vi "BuildingSingleImageGreyLevelDataBase.vi"(6 "Running Index":i32, 8 "error in (no error)":errorcluster, 9 "ConfDB":T1={"NumberOfImages"=0, "NoImages2SaveAroundFreeze"=0, "Path"=path "", "NameOfPartialFile"="", "StartIndex"=0, "NumberOfStdTol"=0, "Detla t (sec)"=0, "Number of images for baseline"=10, "Temperature File Name"="", "Score"=15.0, "Index number of Files"=[], "End Index"=2187}, 10 "Droplet Bounding Box":cluster{"x":sgl, "y":sgl}[][](array[cluster]), 11 "Image Ref In":T2) -> (0 "error out":errorcluster, 1 "Difference in Grey Level":dbl[](array[numeric]), 2 "GreyLevelArray":dbl[](array[numeric]))   [LabVIEW 2013]
doc: "Go over all images and retrieve Grey level of each drop and the difference between the i+1 and i image"
uses:
  <vilib>/vision/Image Controls.llb/IMAQ Image.ctl
  DB/ConfDB.ctl
  DB/DbEnum.ctl
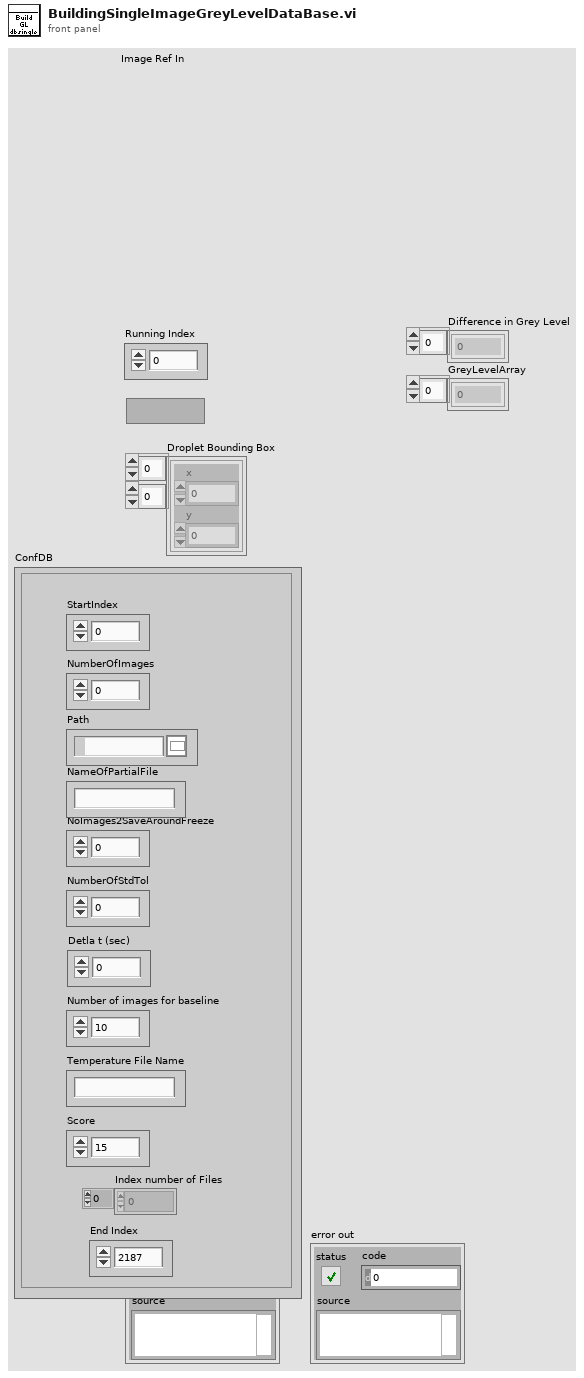
[diagram p1: front panel]
types:
  T1 = typedef "ConfDB.ctl" = cluster{"NumberOfImages":i32, "NoImages2SaveAroundFreeze":i32, "Path":path, "NameOfPartialFile":string, "StartIndex":i32, "NumberOfStdTol":i32, "Detla t (sec)":i32, "Number of images for baseline":i32, "Temperature File Name":string, "Score":dbl, "Index number of Files":i32[], "End Index":i32}
  T2 = typedef "IMAQ Image.ctl" = refnum<image>
  T3 = typedef "DbEnum.ctl" = enum16{"Write DropletDB", "Init", "Insert Detection Result Data", "Insert Grey Level Result", "Insert Baseline Results", "AddFreezeImagesAtCertainDroplet", "UpdateIncludeDroplet", "Insert Freeze Analysis Results", "GetDropDB", "GetNoFreezedDroplets", "GetGreyLevelAndDiff", "GetGreyLevelatIndexTime", "GetDropletsBoundingBox"}
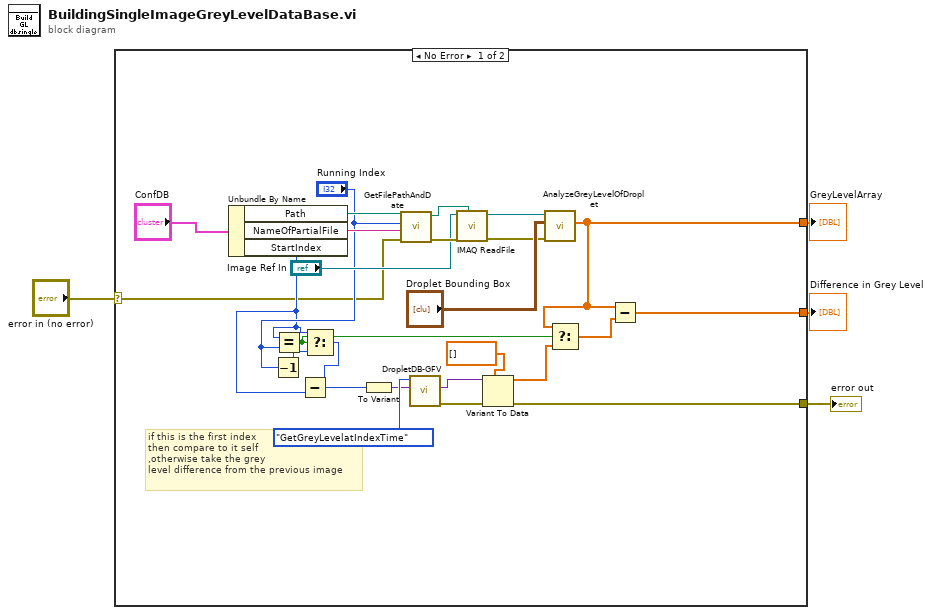
[diagram p0: block diagram]
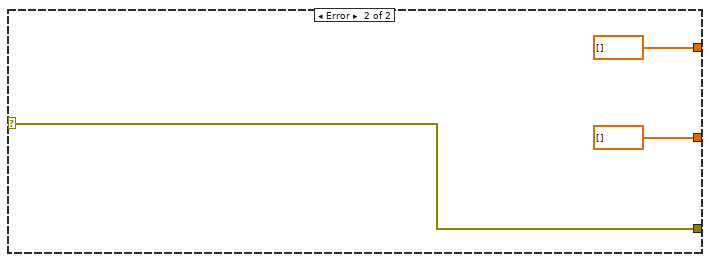
[diagram p2: hidden frame]
diagram:
  n1 = case shown="No Error" "error in (no error)" {
    selector: "error in (no error)" -> [w7 w33]
    tunnel: [w5 w33] -> w3
    tunnel: [w22 dbl[] []] -> w2
    tunnel: [w11 dbl[] [] ("GreyLevelArray")] -> w1
    frame No Error {
      # "if this is the first index\nthen compare to it self\n,otherwise take the grey\nlevel difference from the previous image"
      n2 = Unbundle By Name("ConfDB") -> ("Path"=w25:path, "NameOfPartialFile"=w26:string, "StartIndex"=w14:i32)
      n3 = Decrement(x="Running Index") -> (x-1=w23:i32)
      n4 = Equal?(x=w14, y="Running Index") -> (x = y?=w12:bool)
      n5 = Select(t=w14, s=w12, f=w23) -> (s? t:f=w17:i32)
      n6 = Subtract(x=w17, y=w14) -> (x-y=w13:i32)
      n7 = To Variant(anything=w13) -> (Variant=w18:variant)
      n8 = call "GetFilePathAndDate.vi"("error in (no error)"=w7, "String"=w26, "Index"="Running Index", "Path"=w25) -> ("error out"=w30:errorcluster, "file out"=w8:path)  [unwired: 5 in, 1 out]
      n9 = call "DropletDB-GFV.vi"("Data in"=w18, "Command In"=DbEnum."GetGreyLevelatIndexTime") -> ("error out"=w20:errorcluster, "Data out"=w19:variant)  [unwired: 8 in]
      n10 = call "IMAQ ReadFile"("File Path"=w8, "error in (no error)"=w30, "Image"="Image Ref In") -> ("error out"=w6:errorcluster, "Image Out"=w27:T2)  [unwired: 2 in, 5 out]
      n11 = Variant To Data(error in=w20, type=dbl[] [] ("GreyLevelArray"), Variant=w19) -> (data=w10:dbl[], error out=w5:errorcluster)
      n12 = call "AnalyzeGreyLevelOfDroplet.vi"("error in (no error)"=w6, "Bounding Box"="Droplet Bounding Box", "Image In"=w27) -> ("GreyLevelArray"=w11:dbl[])  [unwired: 6 in, 2 out]
      n13 = Select(t=w11, s=w12, f=w10) -> (s? t:f=w9:dbl[])
      n14 = Subtract(x=w11, y=w9) -> (x-y=w22:dbl[])
    }
    frame Error {
    }
  }
  "error out" <- w3
  "Difference in Grey Level" <- w2
  "GreyLevelArray" <- w1
